vi "Message Handler.vi"(10 "stop notifier":refnum<notifier>, 11 "Messages in":refnum<queue>) -> ()   [LabVIEW 2020, in "Frame Logging.lvlib"]
uses:
  Frame Logging.lvlib
  <vilib>/Utility/SystemLogging/NI_SystemLogging.lvlib
  Shared/loggingThreshold_types.ctl
  Log_Configuration.ctl
  Shared/Frame.ctl
  Logger Interface/Logger Interface.lvclass
  PCAP Frame Logger/PCAP Frame Logger.lvclass
  Message_Request_Action.ctl
  Message_Request.ctl
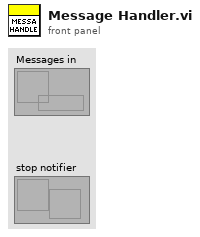
[diagram p1: front panel]
types:
  T1 = typedef "Frame Logging.lvlib/Message_Request.ctl" = cluster{"request":T2, "data":variant}
  T2 = typedef "Frame Logging.lvlib/Message_Request_Action.ctl" = enum16{"Initialize", "Open File", "Log", "Manage Disk", "Stop", "Close File", "Update Configuration"}
  T3 = typedef "Frame.ctl" = cluster{"FwIrigTime":cluster{"TtHigh":u32, "TtLow":u32}, "Payload":u8[], "Lenght":u32}
  T4 = typedef "Frame Logging.lvlib/Log_Configuration.ctl" = cluster{"Log File Directory":string, "Base name":string, "Timestamp":bool, "log thresholds":T5}
  T5 = typedef "loggingThreshold_types.ctl" = cluster{"Segmentation Threshold":dbl, "Disk Space Percentage":dbl, "Check Disk Space":bool, "Segment File":bool, "Segment Files By":u16}
  T6 = enum16{"no action", "close file", "segment file"}
  T7 = cluster{"Logger Interface out":refnum<class "Logger Interface.lvclass">}
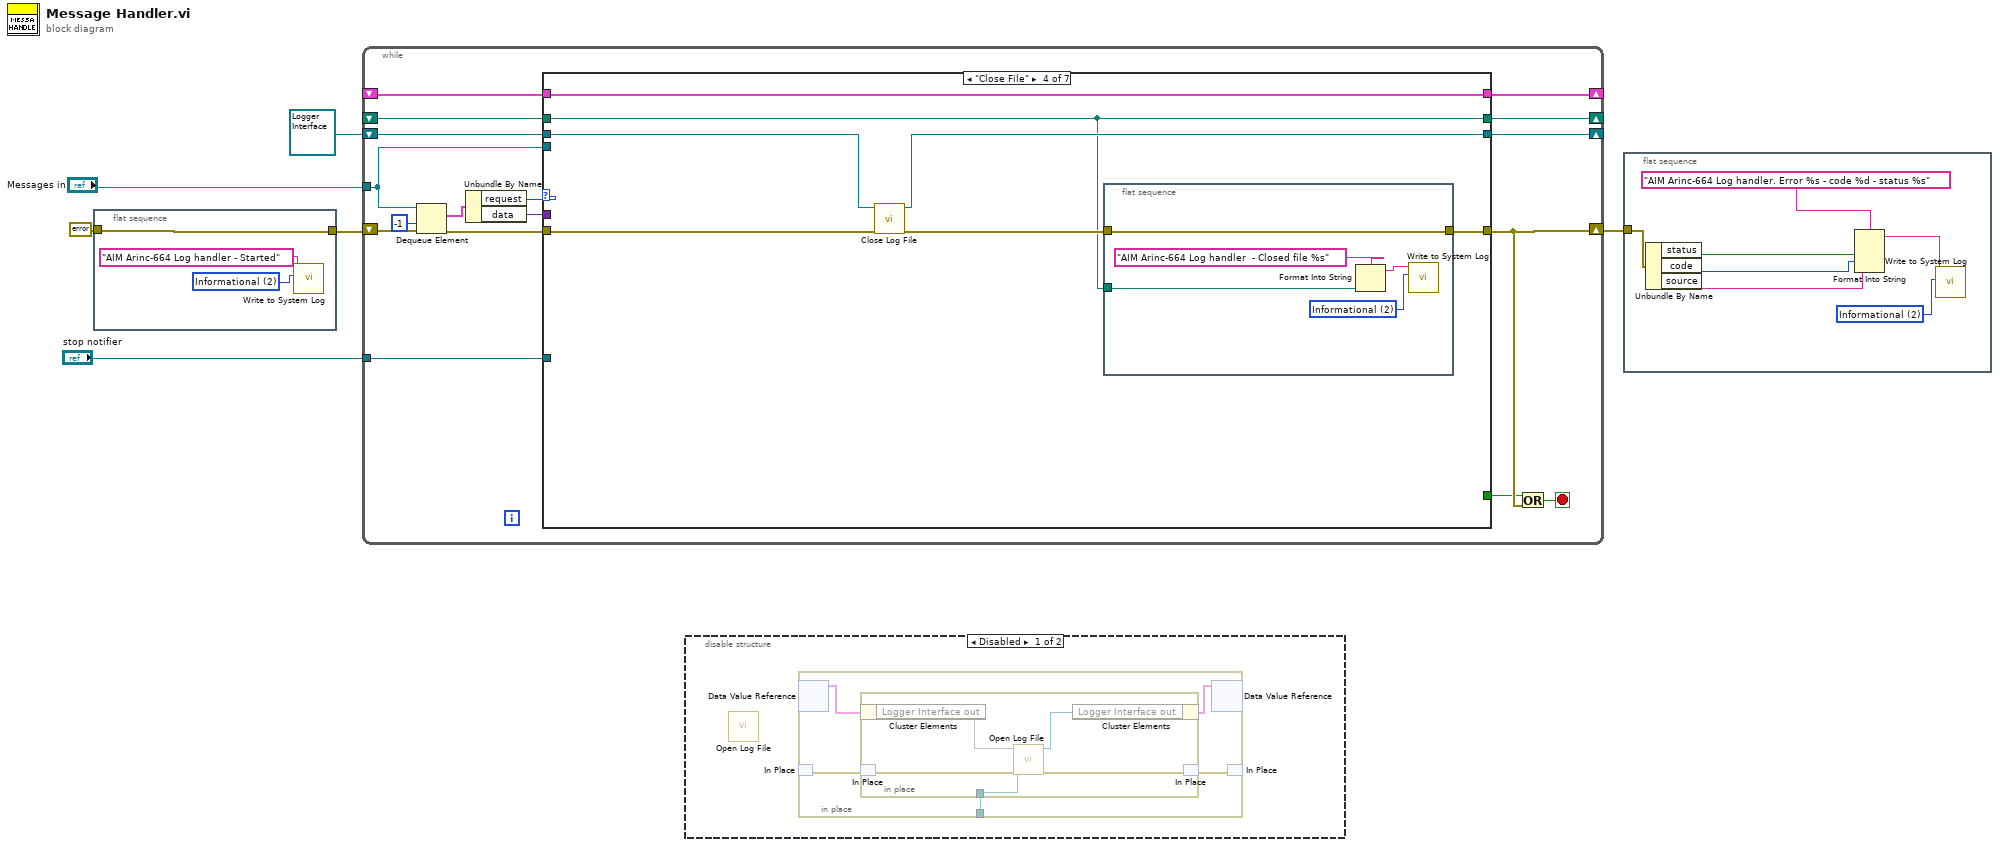
[diagram p0: block diagram]
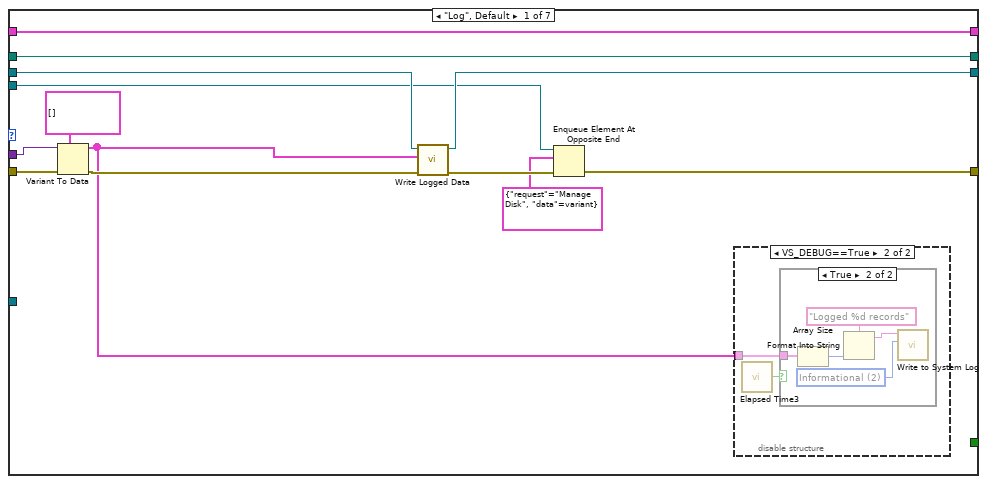
[diagram p3: hidden frame]
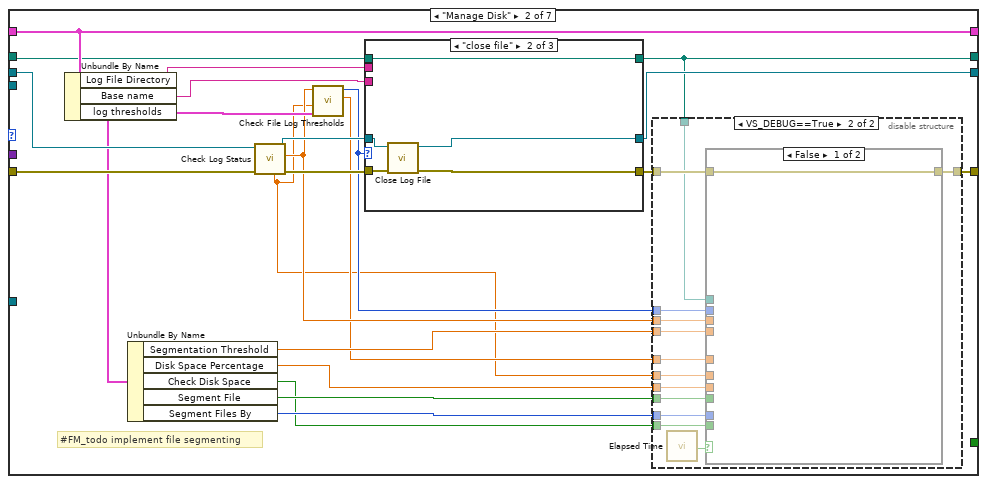
[diagram p6: hidden frame]
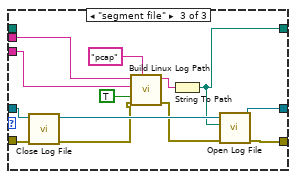
[diagram p8: hidden frame]
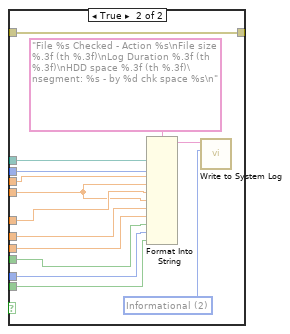
[diagram p10: hidden frame]
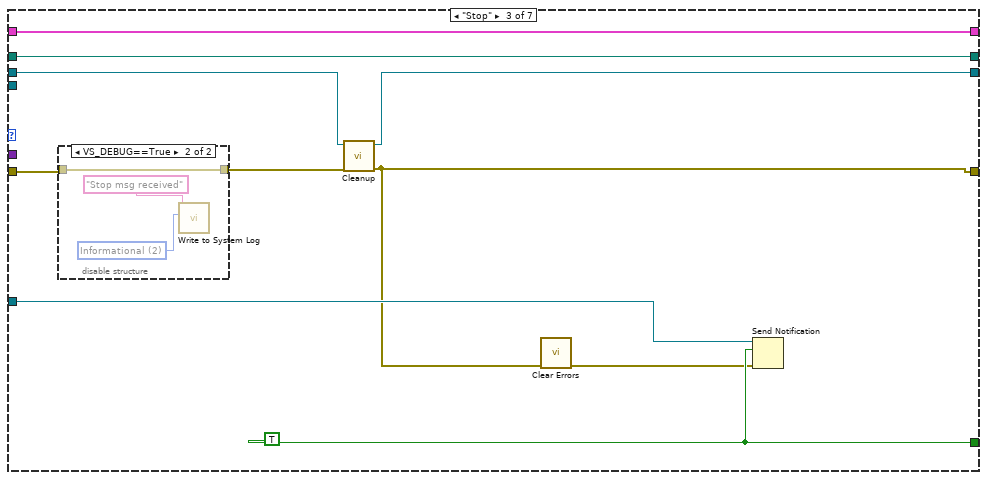
[diagram p11: hidden frame]
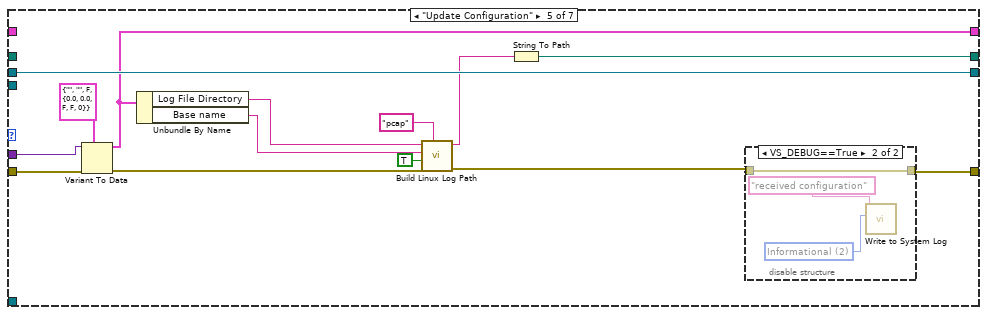
[diagram p13: hidden frame]
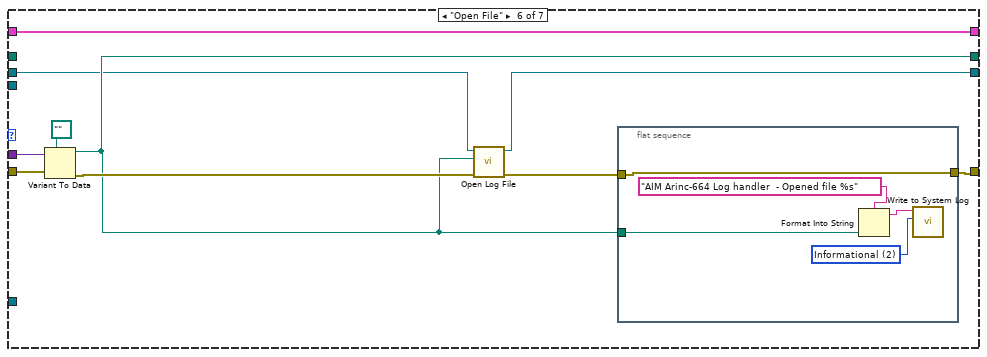
[diagram p15: hidden frame]
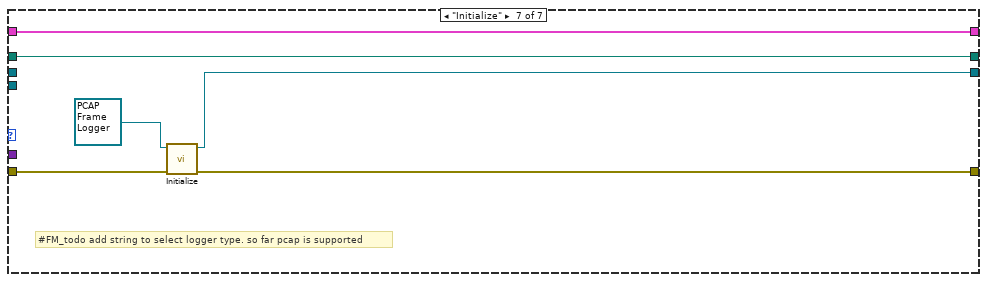
[diagram p16: hidden frame]
diagram:
  n1 = flat-sequence {
    tunnel: errorcluster {"status"=FALSE, "code"=0, "source"=""} ("error in (no error)") -> [w7]
    tunnel: [w7] -> w1
    frame #0 {
      w9 = 2 items=["Error", "Warning", "Informational"] ("severity")
      n2 = call <vilib>:"Write to System Log.vi"("severity"=w9, "message"="AIM Arinc-664 Log handler - Started" ("format string")) -> ()  [unwired: 9 in, 1 out]
    }
  }
  n3 = while {
    tunnel: "Messages in" -> [w10]
    shift-right: [w19] -> w5
    shift-left: w1 -> [w25]
    shift-right: [w17] -> _
    shift-left: _ -> [w16]
    shift-right: [w15] -> _
    shift-left: _ -> [w14]
    tunnel: "stop notifier" -> [w13]
    shift-right: [w12] -> _
    shift-left: refnum<class "Logger Interface.lvclass"> refnum ("Communication Bus Template Interfaces:Implementation.lvlib:Frame Logging.lvlib:Logger Interface.lvclass") -> [w11]
    stop <- w26 stop-if-true
    n4 = Dequeue Element(queue=w10, timeout in ms (-1)=-1, error in (no error)=w25) -> (element=w23:T1, error out=w20:errorcluster)  [unwired: 2 out]
    n5 = Unbundle By Name(w23) -> ("request"=w21:T2, "data"=w22:variant)
    n6 = case shown="\"Close File\"" w21 {
      tunnel: w22 -> [w37 _ _ _ w155 w167 _]
      tunnel: w20 -> [w38 w67 w127 w136 w156 w168 w176]
      tunnel: [w28 w68 w120 w133 w153 w160 w175] -> w19
      tunnel: [_ _ w123 _ _ _ _] -> w18
      tunnel: [w39 w65 w126 w137 w146 w169 w180] -> w17
      tunnel: w16 -> [w39 w65 w126 w137 _ w169 w180]
      tunnel: [w35 w59 w125 w131 w148 w164 w179] -> w15
      tunnel: w14 -> [w35 w60 w125 w131 _ _ w179]
      tunnel: w13 -> [_ _ w124 _ _ _ _]
      tunnel: [w31 w61 w118 w134 w152 w162 w177] -> w12
      tunnel: w11 -> [w32 w62 w121 w135 w152 w163 _]
      tunnel: w10 -> [w30 _ _ _ _ _ _]
      frame "Log", Default {
        n7 = Variant To Data(error in=w38, type=T3[] [] ("Data"), Variant=w37) -> (data=w33:T3[], error out=w34:errorcluster)
        n8 = call-dynamic "Write Logged Data.vi"("error in (no error)"=w34, "Data"=w33, "Logger Interface in"=w32) -> ("error out"=w29:errorcluster, "Logger Interface out"=w31:refnum<class "Logger Interface.lvclass">)  [unwired: 7 in]
        n9 = Enqueue Element At Opposite End(queue=w30, element=T1 {"request"=enum."Manage Disk", "data"=variant}, error in (no error)=w29) -> (error out=w28:errorcluster)  [unwired: 1 in, 2 out]
        n10 = disable-structure shown="VS_DEBUG==True" {
          disable-tunnel: w33 -> [_ w41]
          frame condition #0 (active) {
          }
          frame condition #1 {
            n11 = call "Elapsed Time3"() -> ("Time has Elapsed"=w40:bool)  [unwired: 12 in, 7 out]
            n12 = case shown="True" w40 {
              tunnel: w41 -> [_ w43]
              frame False {
              }
              frame True {
                w46 = 2 items=["Error", "Warning", "Informational"] ("severity")
                n13 = Array Size(array=w43) -> (size(s)=w42:i32)
                n14 = Format Into String(format string="Logged %d records", w42) -> (resulting string=w44:string)  [unwired: 2 in, 1 out]
                n15 = call <vilib>:"Write to System Log.vi"("severity"=w46, "message"=w44) -> ()  [unwired: 9 in, 1 out]
              }
            }
          }
        }
      }
      frame "Manage Disk" {
        # "#FM_todo implement file segmenting"
        n16 = Unbundle By Name(w65) -> ("Log File Directory"=w48:string, "Base name"=w47:string, "log thresholds"=w57:T5)
        n17 = Unbundle By Name(w57) -> ("Segmentation Threshold"=w55:dbl, "Disk Space Percentage"=w52:dbl, "Check Disk Space"=w49:bool, "Segment File"=w51:bool, "Segment Files By"=w50:u16)
        n18 = call-dynamic "Check Log Status.vi"("error in"=w67, "Logger Interface in"=w62) -> ("error out"=w63:errorcluster, "Log file Size MB"=w56:dbl, "Logger Interface out"=w64:refnum<class "Logger Interface.lvclass">, "Hard Drive Space Used (%)"=w53:dbl)  [unwired: 5 in, 1 out]
        n19 = call "Check File Log Thresholds.vi"("log thresholds"=w57, "Hard Drive Space Used (%)"=w53, "Log file Size MB"=w56) -> ("Elapsed Time (s)"=w54:dbl, "action"=w58:T6)  [unwired: 7 in]
        n20 = case shown="\"close file\"" w58 {
          tunnel: w64 -> [w70 w76 w89]
          tunnel: w63 -> [w71 w75 w88]
          tunnel: [w71 w74 w85] -> w66
          tunnel: [w70 w73 w86] -> w61
          tunnel: w60 -> [w69 w72 _]
          tunnel: [w69 w72 w78] -> w59
          tunnel: w48 -> [_ _ w77]
          tunnel: w47 -> [_ _ w82]
          frame "no action", Default {
          }
          frame "close file" {
            n21 = call-dynamic "Close Log File.vi"("error in (no error)"=w75, "Logger Interface in"=w76) -> ("error out"=w74:errorcluster, "Logger Interface out"=w73:refnum<class "Logger Interface.lvclass">)  [unwired: 8 in]
          }
          frame "segment file" {
            n22 = call-dynamic "Close Log File.vi"("error in (no error)"=w88, "Logger Interface in"=w89) -> ("error out"=w81:errorcluster, "Logger Interface out"=w87:refnum<class "Logger Interface.lvclass">)  [unwired: 8 in]
            n23 = call "Build Linux Log Path.vi"("Extension"="pcap", "error in (no error)"=w81, "Timestamp"=TRUE, "Name"=w82, "Log File Directory"=w77) -> ("error out"=w80:errorcluster, "Log File Path"=w79:string)  [unwired: 5 in]
            n24 = String To Path(string=w79) -> (path=w78:path)
            n25 = call-dynamic "Open Log File.vi"("error in (no error)"=w80, "Path"=w78, "Logger Interface in"=w87) -> ("error out"=w85:errorcluster, "Logger Interface out"=w86:refnum<class "Logger Interface.lvclass">)  [unwired: 7 in]
          }
        }
        n26 = disable-structure shown="VS_DEBUG==True" {
          disable-tunnel: w66 -> [_ w102]
          disable-tunnel: [_ w101] -> w68
          disable-tunnel: w59 -> [_ w99]
          disable-tunnel: w58 -> [_ w98]
          disable-tunnel: w56 -> [_ w97]
          disable-tunnel: w55 -> [_ w96]
          disable-tunnel: w54 -> [_ w95]
          disable-tunnel: w53 -> [_ w94]
          disable-tunnel: w52 -> [_ w93]
          disable-tunnel: w51 -> [_ w92]
          disable-tunnel: w50 -> [_ w91]
          disable-tunnel: w49 -> [_ w90]
          frame condition #0 (active) {
          }
          frame condition #1 {
            n27 = call "Elapsed Time"() -> ("Time has Elapsed"=w100:bool)  [unwired: 12 in, 7 out]
            n28 = case shown="False" w100 {
              tunnel: w102 -> [w103 w114]
              tunnel: [w103 w114] -> w101
              tunnel: w99 -> [_ w113]
              tunnel: w98 -> [_ w112]
              tunnel: w97 -> [_ w111]
              tunnel: w96 -> [_ w109]
              tunnel: w95 -> [_ w110]
              tunnel: w94 -> [_ w108]
              tunnel: w93 -> [_ w107]
              tunnel: w92 -> [_ w106]
              tunnel: w91 -> [_ w105]
              tunnel: w90 -> [_ w104]
              frame False {
              }
              frame True {
                w117 = 2 items=["Error", "Warning", "Informational"] ("severity")
                n29 = Format Into String(format string="File %s Checked - Action %s\nFile size %.3f (th %.3f)\nLog Duration %.3f (th %.3f)\nHDD space %.3f (th %.3f)\nsegment: %s - by %d chk space %s\n", w113, w112, w111, w109, w110, w109, w108, w107, w106, w105, w104) -> (resulting string=w115:string)  [unwired: 2 in, 1 out]
                n30 = call <vilib>:"Write to System Log.vi"("severity"=w117, "message"=w115) -> ()  [unwired: 9 in, 1 out]
              }
            }
          }
        }
      }
      frame "Stop" {
        w123 = TRUE
        n31 = disable-structure shown="VS_DEBUG==True" {
          disable-tunnel: w127 -> [_ w129]
          disable-tunnel: [_ w129] -> w122
          frame condition #0 (active) {
          }
          frame condition #1 {
            w130 = 2 items=["Error", "Warning", "Informational"] ("severity")
            n32 = call <vilib>:"Write to System Log.vi"("severity"=w130, "message"="Stop msg received" ("format string")) -> ()  [unwired: 9 in, 1 out]
          }
        }
        n33 = call-dynamic "Cleanup.vi"("error in"=w122, "Logger Interface in"=w121) -> ("error out"=w120:errorcluster, "Logger Interface out"=w118:refnum<class "Logger Interface.lvclass">)  [unwired: 8 in]
        n34 = call <vilib>:"Clear Errors.vi"("error in (no error)"=w120) -> ("error out"=w119:errorcluster)  [unwired: 5 in, 1 out]
        n35 = Send Notification(notification=w123, notifier=w124, error in (no error)=w119) -> ()  [unwired: 2 out]
      }
      frame "Close File" {
        n36 = call-dynamic "Close Log File.vi"("error in (no error)"=w136, "Logger Interface in"=w135) -> ("error out"=w132:errorcluster, "Logger Interface out"=w134:refnum<class "Logger Interface.lvclass">)  [unwired: 8 in]
        n37 = flat-sequence {
          tunnel: w131 -> [w142]
          tunnel: w132 -> [w138]
          tunnel: [w138] -> w133
          frame #0 {
            w141 = 2 items=["Error", "Warning", "Informational"] ("severity")
            n38 = Format Into String(format string="AIM Arinc-664 Log handler  - Closed file %s", w142) -> (resulting string=w139:string)  [unwired: 2 in, 1 out]
            n39 = call <vilib>:"Write to System Log.vi"("severity"=w141, "message"=w139) -> ()  [unwired: 9 in, 1 out]
          }
        }
      }
      frame "Update Configuration" {
        n40 = Variant To Data(error in=w156, type=T4 {"Log File Directory"="", "Base name"="", "Timestamp"=FALSE, "log thresholds"={"Segmentation Threshold"=0.0, "Disk Space Percentage"=0.0, "Check Disk Space"=FALSE, "Segment File"=FALSE, "Segment Files By"=0}} ("log configuration"), Variant=w155) -> (data=w146:T4, error out=w151:errorcluster)
        n41 = Unbundle By Name(w146) -> ("Log File Directory"=w145:string, "Base name"=w144:string)
        n42 = call "Build Linux Log Path.vi"("Extension"="pcap", "error in (no error)"=w151, "Timestamp"=TRUE, "Name"=w144, "Log File Directory"=w145) -> ("error out"=w147:errorcluster, "Log File Path"=w149:string)  [unwired: 5 in]
        n43 = String To Path(string=w149) -> (path=w148:path)
        n44 = disable-structure shown="VS_DEBUG==True" {
          disable-tunnel: w147 -> [_ w158]
          disable-tunnel: [_ w158] -> w153
          frame condition #0 (active) {
          }
          frame condition #1 {
            w159 = 2 items=["Error", "Warning", "Informational"] ("severity")
            n45 = call <vilib>:"Write to System Log.vi"("severity"=w159, "message"="received configuration" ("format string")) -> ()  [unwired: 9 in, 1 out]
          }
        }
      }
      frame "Open File" {
        n46 = Variant To Data(error in=w168, type=path "", Variant=w167) -> (data=w164:path, error out=w165:errorcluster)
        n47 = call-dynamic "Open Log File.vi"("error in (no error)"=w165, "Path"=w164, "Logger Interface in"=w163) -> ("error out"=w161:errorcluster, "Logger Interface out"=w162:refnum<class "Logger Interface.lvclass">)  [unwired: 7 in]
        n48 = flat-sequence {
          tunnel: w164 -> [w174]
          tunnel: w161 -> [w170]
          tunnel: [w170] -> w160
          frame #0 {
            w173 = 2 items=["Error", "Warning", "Informational"] ("severity")
            n49 = Format Into String(format string="AIM Arinc-664 Log handler  - Opened file %s", w174) -> (resulting string=w171:string)  [unwired: 2 in, 1 out]
            n50 = call <vilib>:"Write to System Log.vi"("severity"=w173, "message"=w171) -> ()  [unwired: 9 in, 1 out]
          }
        }
      }
      frame "Initialize" {
        # "#FM_todo add string to select logger type. so far pcap is supported"
        n51 = call-dynamic "Initialize.vi"("error in"=w176, "PCAP Frame Logger in"=refnum<class "PCAP Frame Logger.lvclass"> refnum ("Communication Bus Template Interfaces:Implementation.lvlib:Frame Logging.lvlib:PCAP Frame Logger.lvclass")) -> ("error out"=w175:errorcluster, "PCAP Frame Logger out"=w177:refnum<class "PCAP Frame Logger.lvclass">)  [unwired: 8 in]
      }
    }
    n52 = Or(x=w18, y=w19) -> (x .or. y?=w26:bool)
  }
  n53 = disable-structure shown="Disabled" {
    frame Disabled {
      n54 = call-dynamic "Open Log File.vi"() -> ()  [unwired: 10 in, 2 out]
      n55 = in-place {
        in-place-border: _ -> [w182]
        n56 = in-place-dvr #1() -> (w183:T7)  [unwired: 1 in, 1 out]
        n57 = in-place-match #2() -> (w185:errorcluster)  [unwired: 1 in]
        n58 = in-place {
          in-place-border: w182 -> [w186]
          n59 = in-place-cluster #3(w183) -> ("Logger Interface out"=w190)
          n60 = in-place-match #4(w185) -> (w188:errorcluster)
          n61 = call-dynamic "Open Log File.vi"("error in (no error)"=w188, "Path"=w186, "Logger Interface in"=w190) -> ("error out"=w187:errorcluster, "Logger Interface out"=w189:refnum<class "Logger Interface.lvclass">)  [unwired: 7 in]
          n62 = in-place-cluster #3("Logger Interface out"=w189) -> (w181:cluster{})
          n63 = in-place-match #4(w187) -> (w184:errorcluster)
        }
        n64 = in-place-dvr #1(w181) -> ()  [unwired: 2 out]
        n65 = in-place-match #2(w184) -> ()  [unwired: 1 out]
      }
    }
    frame Enabled {
    }
  }
  n66 = flat-sequence {
    tunnel: w5 -> [w197]
    frame #0 {
      w196 = 2 items=["Error", "Warning", "Informational"] ("severity")
      n67 = Unbundle By Name(w197) -> ("status"=w193:bool, "code"=w192:i32, "source"=w191:string)
      n68 = Format Into String(format string="AIM Arinc-664 Log handler. Error %s - code %d - status %s", w193, w192, w191) -> (resulting string=w194:string)  [unwired: 2 in, 1 out]
      n69 = call <vilib>:"Write to System Log.vi"("severity"=w196, "message"=w194) -> ()  [unwired: 9 in, 1 out]
    }
  }
